vi "Stop Continuous Value (SubVI).vi"(2 "entrée d'erreur":errorcluster, 3 "Refnum VISA en entrée":refnum<visa-resource-name>) -> (0 "sortie d'erreur":errorcluster, 1 "Refnum VISA en sortie":refnum<visa-resource-name>)   [LabVIEW 2017]
doc: "Send charcater by character the commabd to stop continous value.\nMade by Tanguy BOULARD\nTHALES FRANCE"
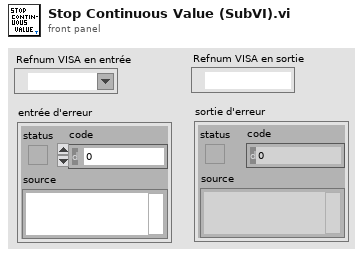
[diagram p1: front panel]
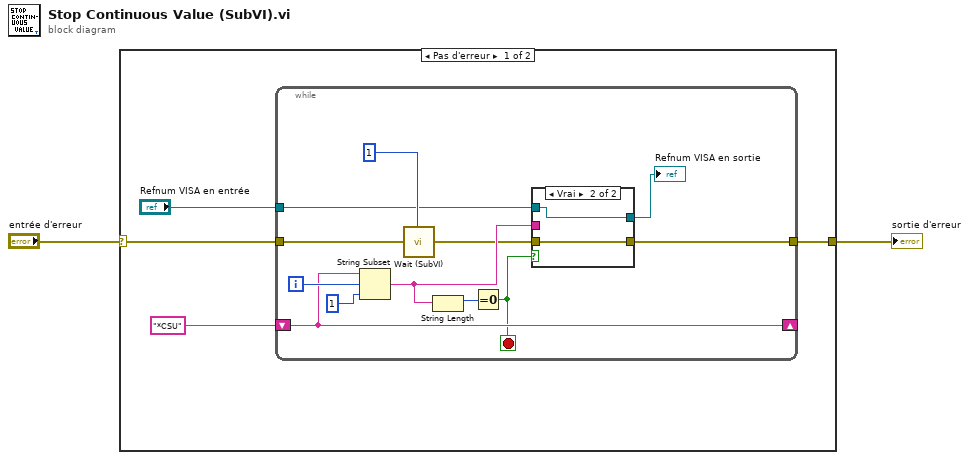
[diagram p0: block diagram]
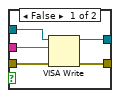
[diagram p2: hidden frame]
diagram:
  n1 = case shown="Pas d'erreur" "entrée d'erreur" {
    selector: "entrée d'erreur" -> [w6 w26]
    tunnel: [w5 w26] -> w2
    frame No Error {
      n2 = while {
        shift-right: [w16] -> _
        shift-left: "*CSU" ("write buffer") -> [w16]
        tunnel: w6 -> [w12]
        tunnel: [w10] -> w5
        tunnel: "Refnum VISA en entrée" -> [w7]
        i -> [w17]
        stop <- w14 stop-if-true
        n3 = String Subset(string=w16, offset (0)=w17, length (rest)=1 ("length (rest)")) -> (substring=w13:string)
        n4 = call "Wait (SubVI).vi"("error in"=w12, "attente (ms)"=u32 1 ("delay")) -> ("error out"=w11:errorcluster)  [unwired: 25 in]
        n5 = String Length(string=w13) -> (length=w15:i32)
        n6 = Equal To 0?(x=w15) -> (x = 0?=w14:bool)
        n7 = case shown="Vrai" w14 {
          tunnel: w13 -> [w23 _]
          tunnel: [w22 w24] -> w9
          tunnel: w11 -> [w21 w25]
          tunnel: [w20 w25] -> w10
          tunnel: w7 -> [w19 w24]
          frame False {
            n8 = VISA Write(VISA resource name=w19, write buffer=w23, error in (no error)=w21) -> (VISA resource name out=w22:refnum<visa-resource-name>, error out=w20:errorcluster)  [unwired: 1 out]
          }
          frame True {
          }
        }
        "Refnum VISA en sortie" <- w9
      }
    }
    frame Error {
    }
  }
  "sortie d'erreur" <- w2
